vi "Create.vi"(7 "Size":cluster{"Width":u16, "Height":u16}={"Width"=32, "Height"=32}, 8 "error in (no error)":errorcluster, 10 "Index (42)":i32=42, 11 "Listbox":refnum<vi>) -> (0 "error out":errorcluster, 3 "Listbox Icon Canvas out":refnum<class "Listbox Icon Canvas.lvclass">)   [LabVIEW 2023, in "Font Glyph Drawer Interface.lvlib" / "Listbox Icon Canvas.lvclass"]
uses:
  Listbox Icon Canvas.lvclass
  Listbox Icon Canvas.lvclass/Listbox Icon Canvas.ctl
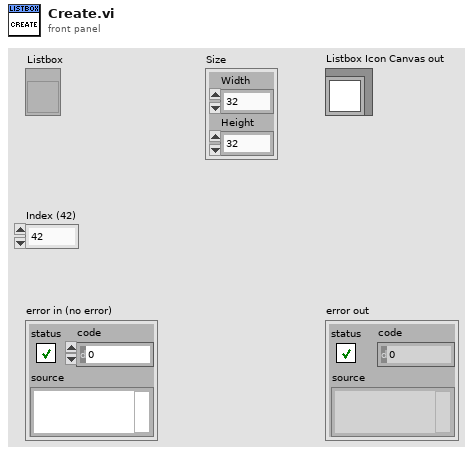
[diagram p1: front panel]
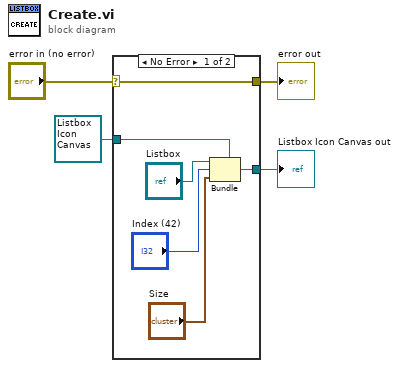
[diagram p0: block diagram]
diagram:
  n1 = case shown="No Error" "error in (no error)" {
    selector: "error in (no error)" -> [w9 w12]
    tunnel: [w9 w12] -> w3
    tunnel: [w8 w11] -> w1
    tunnel: refnum<class "Listbox Icon Canvas.lvclass"> refnum ("Listbox Icon Canvas in") -> [w10 w11]
    frame No Error {
      n2 = Bundle(cluster=w10, "Listbox", "Index (42)", "Size") -> (w8:refnum<class "Listbox Icon Canvas.lvclass">)
    }
    frame Error {
    }
  }
  "error out" <- w3
  "Listbox Icon Canvas out" <- w1
